vi "jsonTest.vi"() -> ()   [LabVIEW 2019]
uses:
  System Explorer/FOM/_typedefs/interaction_json_type.ctl
  System Explorer/HLA Custom Device System Explorer.lvlib
panel:
  out "value 2":T1[](array[typedef])
  out "value":T2(array[cluster])
  in  "JSON string 3":string
  out "JSON string 2":string
  in  "interaction":T2(array[cluster])
  out "JSON string":string
  in  "parameters":cluster{"name":string, "type":string}[](array[cluster])
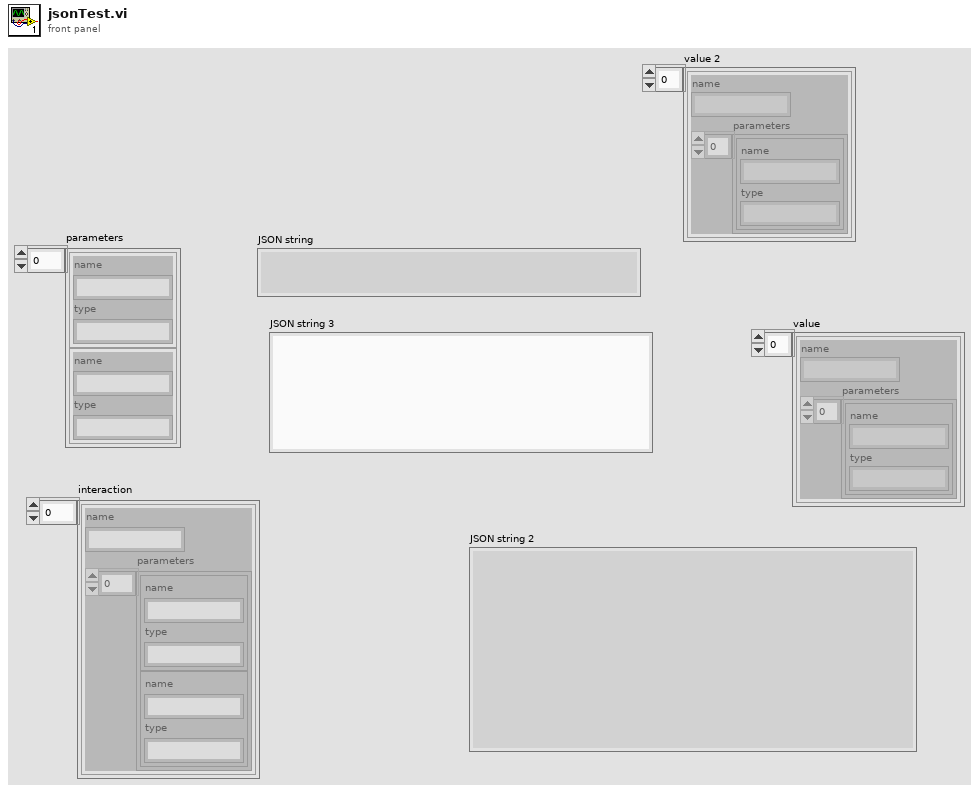
[diagram p1: front panel]
types:
  T1 = typedef "HLA Custom Device System Explorer.lvlib/interaction_json_type.ctl" = cluster{"name":string, "parameters":cluster{"name":string, "type":string}[]}
  T2 = cluster{"name":string, "parameters":cluster{"name":string, "type":string}[]}[]
  T3 = cluster{"name":string, "attributes":cluster{"name":string, "type":string}[]}[]
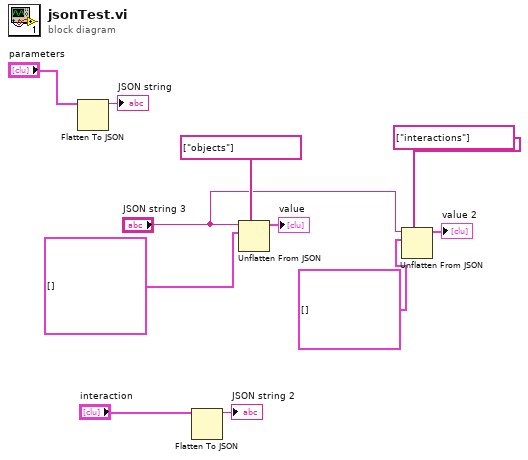
[diagram p0: block diagram]
diagram:
  n1 = Flatten To JSON(anything="parameters") -> (JSON string=→"JSON string":string)  [unwired: 2 in, 1 out]
  n2 = Flatten To JSON(anything="interaction") -> (JSON string=→"JSON string 2":string)  [unwired: 2 in, 1 out]
  n3 = Unflatten From JSON(path=string[] ["objects"], JSON string="JSON string 3", type and defaults=T3 [] ("interaction")) -> (value=→"value":T3)  [unwired: 4 in, 1 out]
  n4 = Unflatten From JSON(path=string[] ["interactions"], JSON string="JSON string 3", type and defaults=T2 [] ("interaction")) -> (value=→"value 2":T2)  [unwired: 4 in, 1 out]
